vi "Valve Map Port Mapping.vi"(8 "Action":T3=enum."Set", 9 "Allowed In Standby?":bool[](array[boolean]), 10 "Solenoid Port List":u8[](array[numeric]), 11 "Valve List":T2[](array[typedef])) -> (2 "Mapping List":T1[](array[typedef]))   [LabVIEW 2015]
uses:
  Valve Port Mapping Action.ctl
  Valve Name Enum.ctl
  Valve Port Mapping.ctl
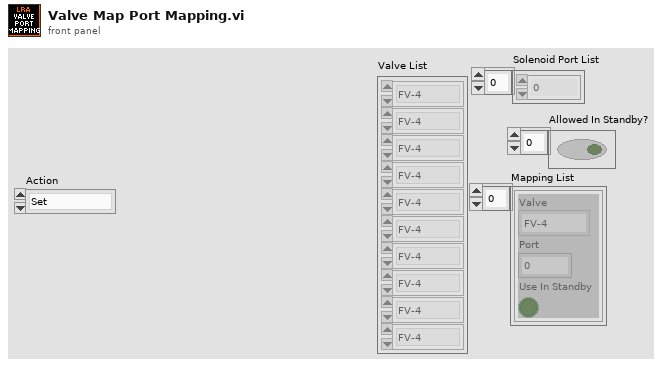
[diagram p1: front panel]
types:
  T1 = typedef "Valve Port Mapping.ctl" = cluster{"Valve":T2, "Port":u8, "Use In Standby":bool}
  T2 = typedef "Valve Name Enum.ctl" = enum16{"FV-4", "FV-3", "FV-2", "OV-4", "OV-3", "OV-2", "NV-2"}
  T3 = typedef "Valve Port Mapping Action.ctl" = enum16{"Get", "Set"}
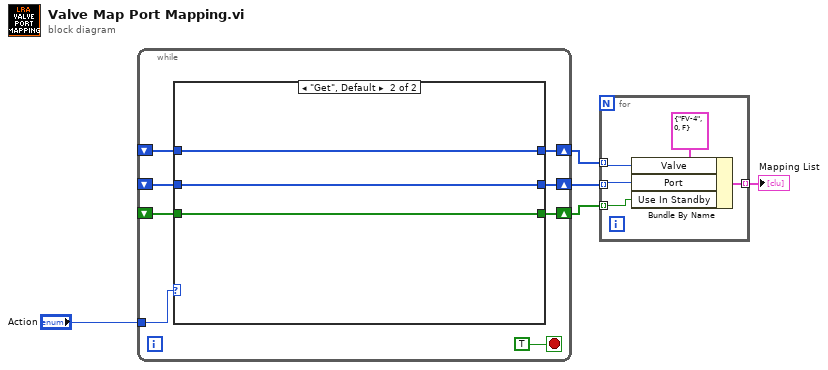
[diagram p0: block diagram]
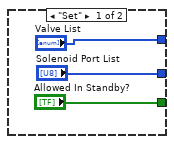
[diagram p2: hidden frame]
diagram:
  n1 = while {
    tunnel: "Action" -> [w12]
    shift-right: [w11] -> w2
    shift-left: _ -> [w8]
    shift-right: [w10] -> w3
    shift-left: _ -> [w7]
    shift-right: [w9] -> w4
    shift-left: _ -> [w6]
    stop <- TRUE stop-if-true
    n2 = case shown="\"Get\", Default" w12 {
      tunnel: ["Valve List" w19] -> w11
      tunnel: ["Solenoid Port List" w18] -> w10
      tunnel: ["Allowed In Standby?" w17] -> w9
      tunnel: w8 -> [_ w19]
      tunnel: w7 -> [_ w18]
      tunnel: w6 -> [_ w17]
      frame "Set" {
      }
      frame "Get", Default {
      }
    }
  }
  n3 = for {
    tunnel: w4 -> [w21] mode=indexing
    tunnel: w3 -> [w22] mode=indexing
    tunnel: w2 -> [w23] mode=indexing
    tunnel: [w20] -> w1 mode=indexing
    n4 = Bundle By Name(cluster=T1 {"Valve"=enum."FV-4", "Port"=0, "Use In Standby"=FALSE} ("Cluster"), "Valve"=w23, "Port"=w22, "Use In Standby"=w21) -> (w20:T1)
  }
  "Mapping List" <- w1
